vi "cleanBG.vi"(8 "error in (no error)":errorcluster, 10 "Table in":refnum<vi>, 11 "reference in":refnum<class "Project Panels.lvclass">) -> (0 "error out":errorcluster, 3 "reference out":refnum<class "Project Panels.lvclass">)   [LabVIEW 2015, in "Project Panels.lvclass"]
uses:
  Project Panels.lvclass
  APP/excelFile_class/fileType.ctl
  SYS/File Controller_llb/File Controller.lvclass
  APP/excelFile_class/excelFile.lvclass
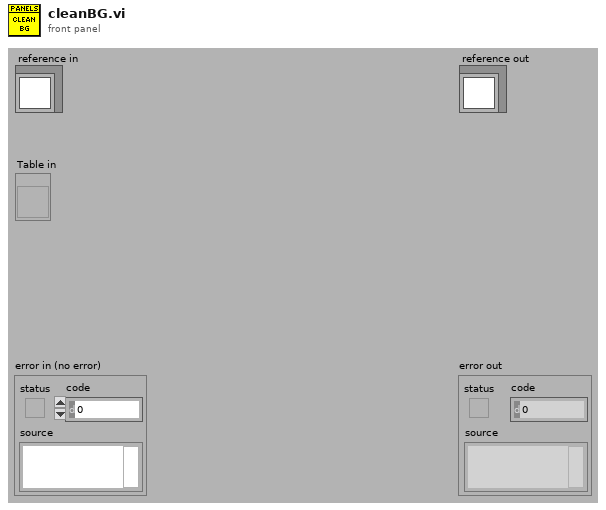
[diagram p1: front panel]
types:
  T1 = typedef "excelFile.lvclass/fileType.ctl" = enum16{"devices", "items", "partsTracking"}
  T2 = typedef "Project Panels.lvclass/ObjectAttributesRef.ctl" = refnum<data-value>
  T3 = typedef "Project Panels.lvclass/ObjectAttributes.ctl" = cluster{"MyAttribute":dbl, "device_controller_ref":refnum<class "Devices Controller.lvclass">, "file_controller_ref":refnum<class "File Controller.lvclass">, "item_controller_ref":refnum<class "Items Controller.lvclass">, "item_tables":cluster{"checkIN":string[][], "checkOUT":string[][], "storage":string[][]}, "quickbook_table":cluster{"notes":string[][]}, "notification_controller_ref":refnum<class "Notification Controller.lvclass">, "partstracking_controller_ref":refnum<class "PartsTracking Controller.lvclass">, "product_tables":cluster{"k4b2":string[][], "fitmate":string[][], "RMR":string[][], "CPET":string[][], "BP":string[][], "PP":string[][], "k5":string[][], "bb-pft":string[][]}, "rowsColour":u32[]}
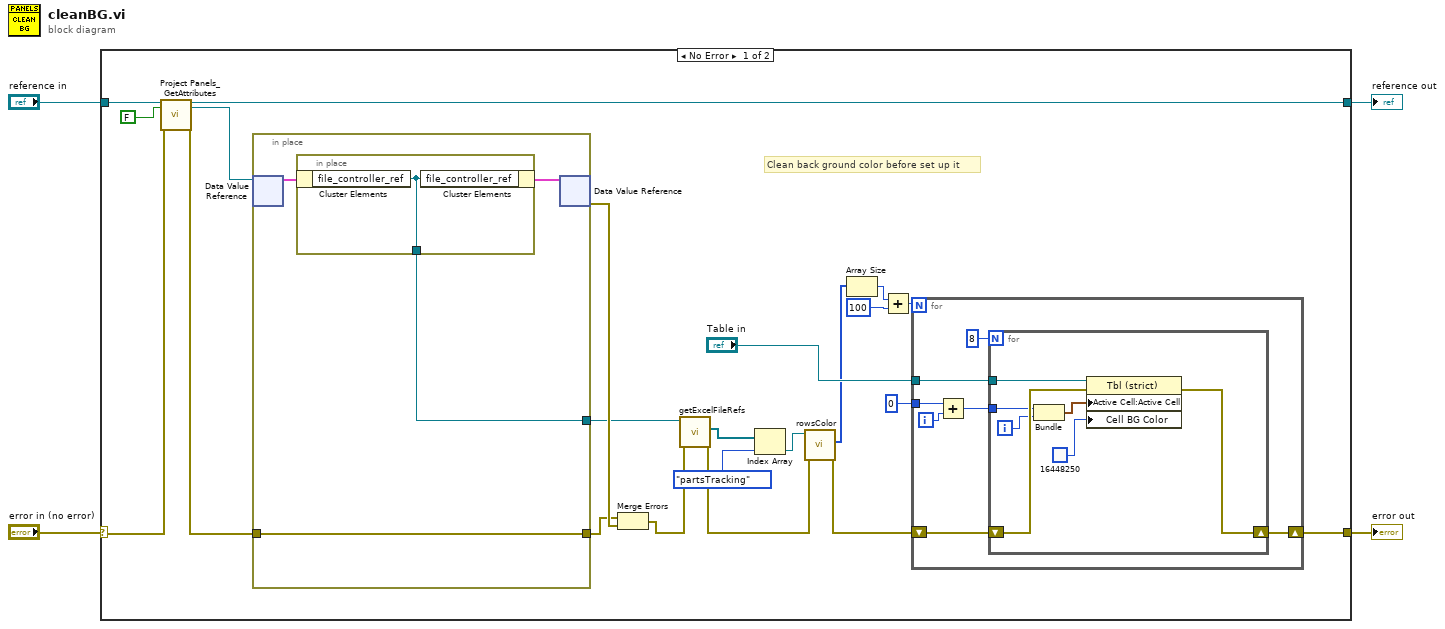
[diagram p0: block diagram]
diagram:
  n1 = case shown="No Error" "error in (no error)" {
    selector: "error in (no error)" -> [w22 w47]
    tunnel: [w10 w47] -> w3
    tunnel: [w20 w46] -> w1
    tunnel: "reference in" -> [w24 w46]
    frame No Error {
      # "Clean back ground color before set up it"
      n2 = call "Project Panels_GetAttributes.vi"("reference in"=w24, "return data? (T)"=FALSE, "error in (no error)"=w22) -> ("reference out"=w20:refnum<class "Project Panels.lvclass">, "attributes ref"=w19:T2, "error out"=w21:errorcluster)  [unwired: 13 in, 1 out]
      n3 = in-place {
        in-place-border: w21 -> [w42]
        in-place-border: [w42] -> w25
        in-place-border: [w41] -> w18
        n4 = in-place-dvr #1(w19) -> (w43:T3)  [unwired: 1 out]
        n5 = in-place {
          in-place-border: [w45] -> w41
          n6 = in-place-cluster #2(w43) -> ("file_controller_ref"=w45:refnum<class "File Controller.lvclass">)
          n7 = in-place-cluster #2("file_controller_ref"=w45) -> (w44:T3)
        }
        n8 = in-place-dvr #1(w44) -> (w26:errorcluster)  [unwired: 1 out]
      }
      n9 = Merge Errors(w25, w26) -> (w17:errorcluster)
      n10 = call "getExcelFileRefs.vi"("error in (no error)"=w17, "reference in"=w18) -> ("error out"=w13:errorcluster, "excelFile_refs"=w16:refnum<class "excelFile.lvclass">[])  [unwired: 7 in, 1 out]
      n11 = Index Array(array=w16, index=fileType."partsTracking" ("fileType")) -> (element=w14:refnum<class "excelFile.lvclass">)
      n12 = call "rowsColor.vi"("error in (no error)"=w13, "reference in"=w14) -> ("error out"=w11:errorcluster, "rowsColor"=w8:u32[])  [unwired: 7 in, 1 out]
      n13 = Array Size(array=w8) -> (size(s)=w7:i32)
      n14 = Add(x=w7, y=100) -> (x+y=w5:i32)
      n15 = for {
        N: w5 -> [_]
        tunnel: "Table in" -> [w31]
        shift-right: [w32] -> w10
        shift-left: w11 -> [w33]
        tunnel: 0 -> [w29]
        i -> [w28]
        n16 = Add(x=w29, y=w28) -> (x+y=w27:i32)
        n17 = for {
          N: 8 -> [_]
          shift-right: [w39] -> w32
          shift-left: w33 -> [w40]
          tunnel: w27 -> [w37]
          tunnel: w31 -> [w38]
          i -> [w36]
          n18 = Bundle(w37, w36) -> (w35:cluster{i32, i32})  [unwired: 1 in]
          n19 = property on="Property Node" class="Tbl (strict)"(reference=w38, error in=w40, "Active Cell:Active Cell"=w35, "Cell BG Color"=u32 16448250) -> (error out=w39:errorcluster)  [unwired: 1 out]
        }
      }
    }
    frame Error {
    }
  }
  "error out" <- w3
  "reference out" <- w1
